vi "CRYStepSetup Global.vi"() -> ()   [LabVIEW 2013]
panel:
  in  "Load from AddStep":bool
  in  "Custom VI Insert":bool
  in  "ApplybyOKCancel":bool
  in  "Step Setup Exist":bool
  in  "sStepEditorName":string
  in  "Step Setup Clicked":bool
  in  "cMsgStepSetup":T1
  in  "sStepNameOld":string
  in  "cStep":T2
  in  "StepVIEWSubVIRef":refnum<vi>
  in  "nStepVINo":i32
  in  "sStepName":string
  in  "Step SubVI Ref":refnum<vi>
  in  "Step Save Finish":bool
  in  "Step SetUp Ref":refnum<vi>
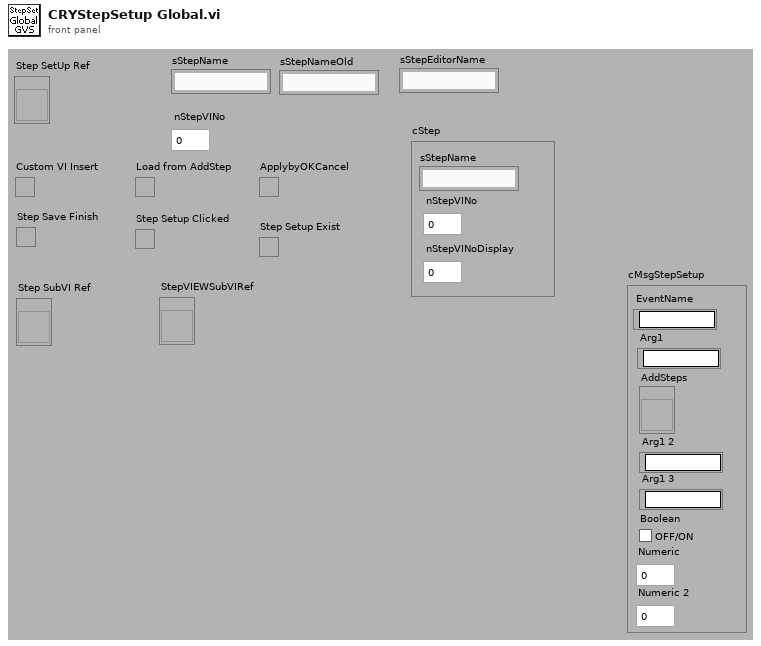
[diagram p1: front panel]
types:
  T1 = cluster{"EventName":string, "Arg1":string, "Numeric":u16, "Numeric 2":u16, "AddSteps ":refnum<vi>, "Arg1 2":string, "Arg1 3":string, "Boolean":bool}
  T2 = cluster{"sStepName":string, "nStepVINo":i32, "nStepVINoDisplay":i32}
diagram:
